vi "emi_ Is Error state.vi"(14 "error in (no error)":errorcluster) -> (3 "error out":errorcluster, 8 "Error State":enum16{"Non", "Warning", "Error"}(ring))   [LabVIEW 2011]
doc: "Extracts teh error status from error cluster,\n \n\nSaves Diagram space at teh expence of execution speed."
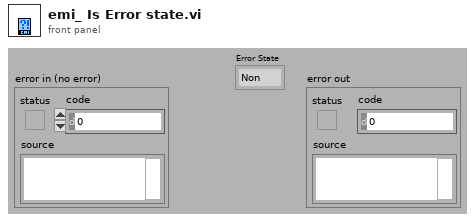
[diagram p1: front panel]
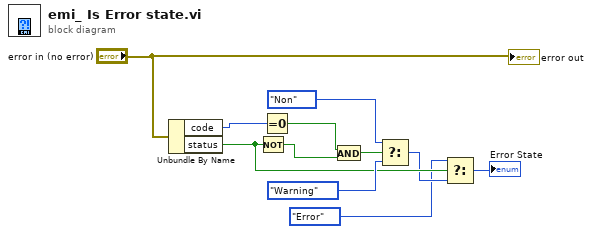
[diagram p0: block diagram]
diagram:
  n1 = Unbundle By Name("error in (no error)") -> ("code"=w10:i32, "status"=w4:bool)
  n2 = Not(x=w4) -> (.not. x?=w8:bool)
  n3 = Equal To 0?(x=w10) -> (x = 0?=w9:bool)
  n4 = And(x=w9, y=w8) -> (x .and. y?=w7:bool)
  n5 = Select(t=enum16{"Non", "Warning", "Error"}."Non", s=w7, f=enum16{"Non", "Warning", "Error"}."Warning") -> (s? t:f=w3:enum16{"Non", "Warning", "Error"})
  n6 = Select(t=enum16{"Non", "Warning", "Error"}."Error", s=w4, f=w3) -> (s? t:f=→"Error State":enum16{"Non", "Warning", "Error"})
  "error out" <- "error in (no error)"
